vi "Dequeue all update control strings, remove duplicates.vi"(8 "error in (no error)":errorcluster, 11 "Fiber Auto Collimation panel":refnum<class "Fiber Auto Collimation panel.lvclass">) -> (0 "error out":errorcluster, 3 "Controls to update":string[](array[string]))   [LabVIEW 2018]
doc: "De-queues all strings previously sent to the \"update controls\" queue, and removes any duplicates or blank strings. The original queue order is preserved."
uses:
  Panels/Fiber Auto Collimation panel.lvclass
  References/Fiber Auto Collimation References.lvclass
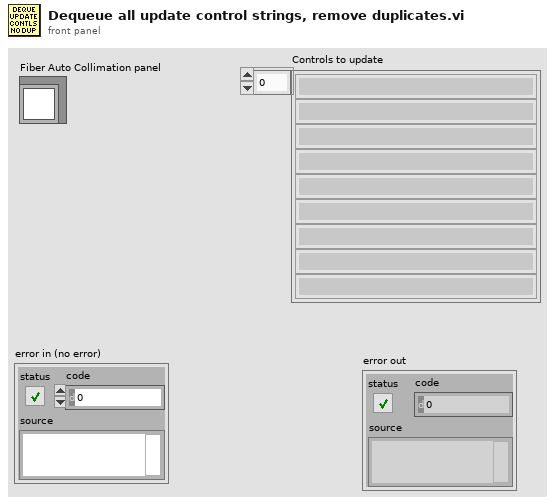
[diagram p1: front panel]
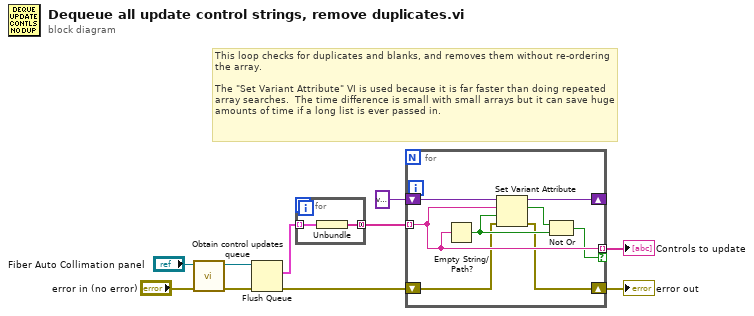
[diagram p0: block diagram]
diagram:
  # "This loop checks for duplicates and blanks, and removes them without re-ordering the array.\n\nThe \"Set Variant Attribute\" VI is used because it is far faster than doing repeated array searches.  The time difference is small with small arrays but it can save huge amounts of time if a long list is ever passed in."
  n1 = call "Obtain control updates queue.vi"("error in (no error)"="error in (no error)", "Fiber Auto Collimation panel"="Fiber Auto Collimation panel") -> ("error out"=w9:errorcluster, "Update control(s) queue out"=w8:refnum<queue>)  [unwired: 8 in]
  n2 = Flush Queue(queue=w8, error in (no error)=w9) -> (remaining elements=w7:cluster{string[]}[], error out=w2:errorcluster)  [unwired: 1 out]
  n3 = for {
    tunnel: w7 -> [w12] mode=indexing
    tunnel: [w11] -> w6 mode=concatenating
    n4 = Unbundle(w12) -> (w11:string[])
  }
  n5 = for {
    tunnel: w6 -> [w18] mode=indexing
    shift-right: [w19] -> _
    shift-left: variant -> [w20]
    tunnel: [w18] -> w4 mode=indexing if=w16
    shift-right: [w13] -> w1
    shift-left: w2 -> [w14]
    n6 = Empty String/Path?(string/path=w18) -> (empty?=w15:bool)
    n7 = Set Variant Attribute(Variant=w20, name=w18, value=w15, error in=w14) -> (Variant out=w19:variant, replaced=w17:bool, error out=w13:errorcluster)
    n8 = Not Or(1:w15, 2:w17) -> (0:w16:bool)
  }
  "error out" <- w1
  "Controls to update" <- w4
